vi "Display Menu.vi"(8 "Startup Menu?(F)":bool, 9 "Display Rules?(F)":bool, 10 "Reference In":refnum<vi>, 11 "Internal Data In":T1) -> (3 "Internal a Out":T1)   [LabVIEW 2025]
uses:
  Internal Data.ctl
  Collision Box.ctl
  <vilib>/picture/picture.llb/imagedata.ctl
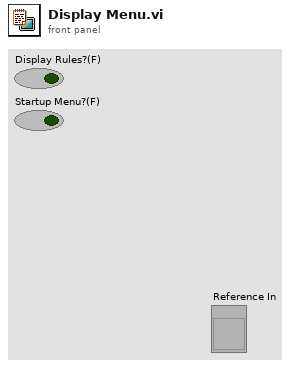
[diagram p1: front panel]
types:
  T1 = typedef "Internal Data.ctl" = cluster{"Core":cluster{"Current VI Reference":refnum<vi>, "Close Panel on Exit?":bool}, "Collision Box":T2, "Walls":cluster{"[0]":T3, "[1]":T3, "[2]":T3, "[3]":T3, "[4]":T3, "[5]":T3, "[6]":T3, "[7]":T3, "[8]":T3}, "Floor":T3, "Gates":cluster{"[0]":T3, "[1]":T3, "[2]":T3, "[3]":T3, "[4]":T3, "[5]":T3, "[6]":T3, "[7]":T3, "[8]":T3}, "Gate Condition":bool[], "Level":i32, "Score":i32, "Player Image":T3, "Display Font":cluster{"Font Name:":string, "Size":i16, "Strikeout?":bool, "Italic?":bool, "Underline?":bool, "Outline?":bool, "Shadow?":bool, "Bold?":bool}, "Menu Image":T3, "Menu Button Image":T3, "Menu Selected Image":T3, "Menu Selection":i32, "Player Name":string, "Menu Wall Image":T3}
  T2 = typedef "Collision Box.ctl" = cluster{"left":i16, "top":i16, "right":i16, "bottom":i16}
  T3 = typedef "imagedata.ctl" = cluster{"image type":i32, "image depth":i32, "image":u8[], "mask":u8[], "colors":u32[], "Rectangle":cluster{"left":i16, "top":i16, "right":i16, "bottom":i16}}
  T4 = enum16{"User-specified Font", "Application Font", "System Font", "Dialog Font"}
  T5 = cluster{"left":i16, "top":i16, "right":i16, "bottom":i16}
  T6 = cluster{"horizontal":enum16{"left", "center", "right"}, "vertical":enum16{"top", "center", "bottom"}}
  T7 = cluster{"Font Name:":string, "Size":i16, "Strikeout?":bool, "Italic?":bool, "Underline?":bool, "Outline?":bool, "Shadow?":bool, "Bold?":bool}
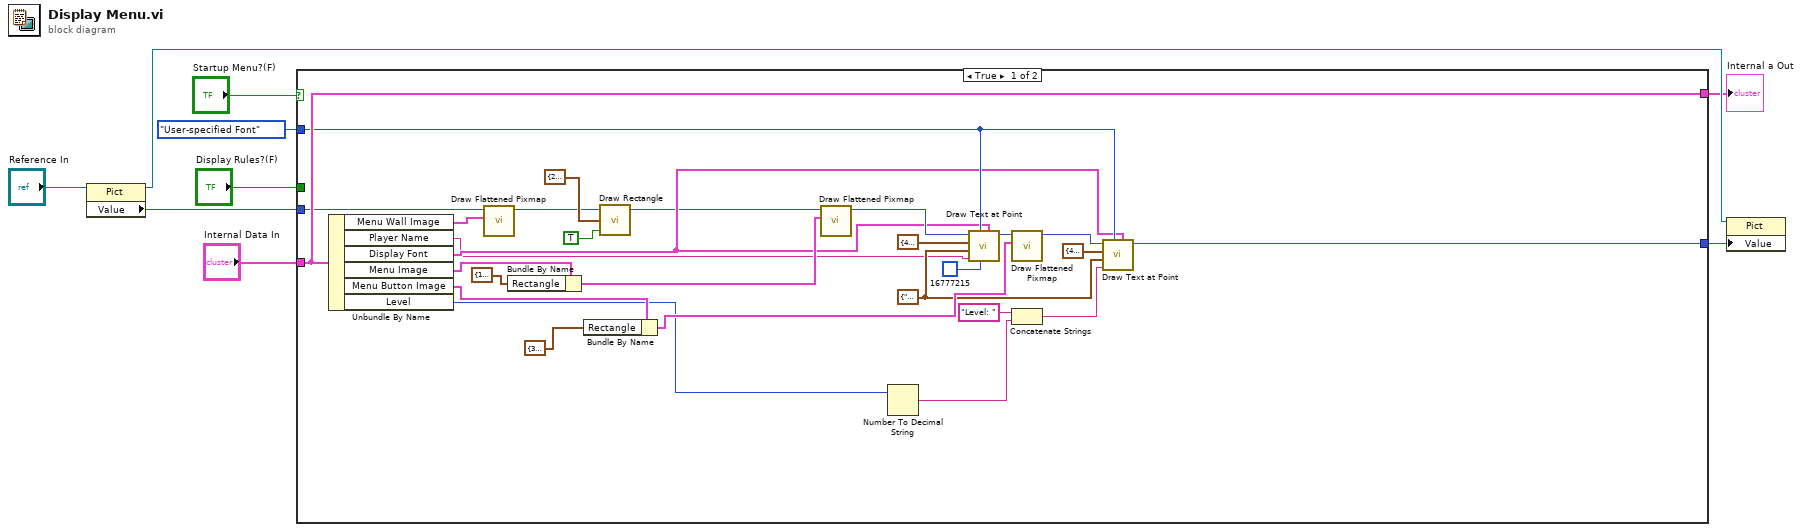
[diagram p0: block diagram]
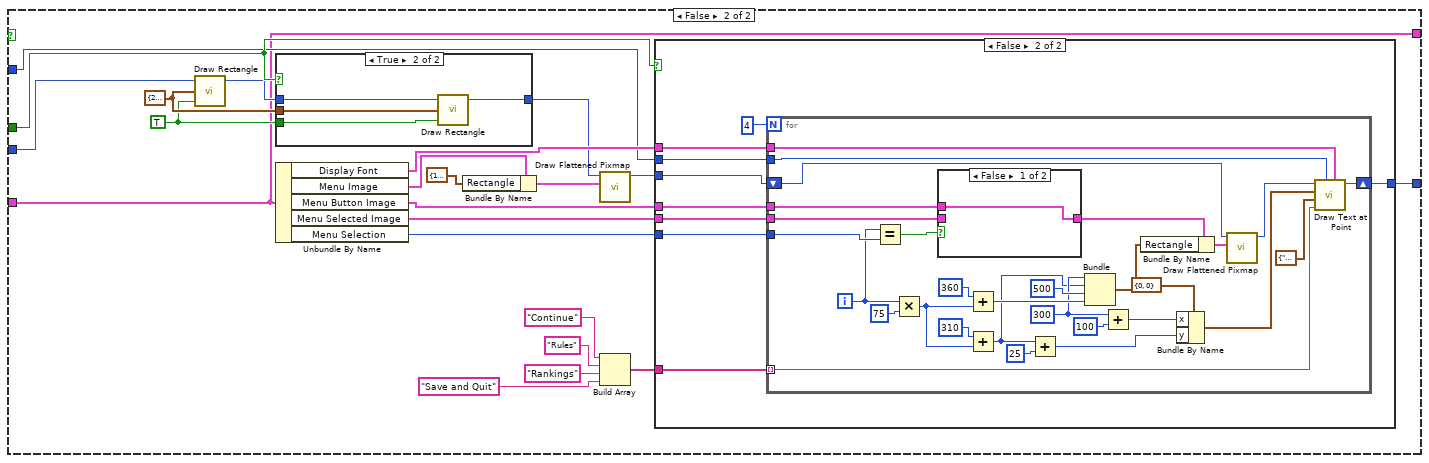
[diagram p2: hidden frame]
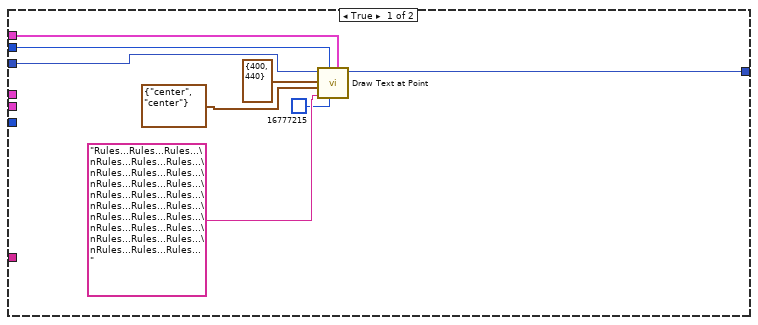
[diagram p3: hidden frame]
diagram:
  n1 = property on="Property Node" class="Pict"(reference="Reference In") -> (reference out=w7:refnum<vi>, "Value"=w6:picture)  [unwired: 1 in, 1 out]
  n2 = case shown="True" "Startup Menu?(F)" {
    tunnel: [w25 w53] -> w9
    tunnel: w6 -> [w15 w51]
    tunnel: "Display Rules?(F)" -> [_ w49]
    tunnel: "Internal Data In" -> [w34 w38]
    tunnel: [w34 w38] -> w1
    tunnel: T4."User-specified Font" ("desired font(Application)") -> [w24 w44]
    frame True {
      w22 = T6 {"horizontal"=enum."center", "vertical"=enum."center"} ("alignment(left, top)")
      n3 = Unbundle By Name(w34) -> ("Menu Wall Image"=w14:T3, "Player Name"=w16:string, "Display Font"=w23:T7, "Menu Image"=w36:T3, "Menu Button Image"=w32:T3, "Level"=w20:i32)
      n4 = call <vilib>:"Draw Flattened Pixmap.vi"("image data"=w14, "picture"=w15) -> ("new picture"=w11:picture)  [unwired: 7 in]
      n5 = Bundle By Name(cluster=w36, "Rectangle"=T5 {"left"=150, "top"=300, "right"=650, "bottom"=815}) -> (w35:T3)
      n6 = Bundle By Name(cluster=w32, "Rectangle"=T5 {"left"=300, "top"=600, "right"=500, "bottom"=650}) -> (w31:T3)
      n7 = call <vilib>:"Draw Rectangle.vi"("picture"=w11, "rect"=T5 {"left"=200, "top"=350, "right"=600, "bottom"=800} ("Rectangle"), "fill?(F)"=TRUE) -> ("new picture"=w10:picture)  [unwired: 6 in]
      n8 = call <vilib>:"Draw Flattened Pixmap.vi"("image data"=w35, "picture"=w10) -> ("new picture"=w30:picture)  [unwired: 7 in]
      n9 = Number To Decimal String(number=w20) -> (decimal integer string=w19:string)  [unwired: 1 in]
      n10 = call <vilib>:"Draw Text at Point.vi"("[user-specified font]"=w23, "text color(black)"=u32 16777215, "desired font(Application)"=w24, "text"=w16, "alignment(left, top)"=w22, "origin"=cluster{"x":i16, "y":i16} {"x"=400, "y"=550}, "picture"=w30) -> ("new picture"=w29:picture)  [unwired: 3 in, 1 out]
      n11 = call <vilib>:"Draw Flattened Pixmap.vi"("image data"=w31, "picture"=w29) -> ("new picture"=w26:picture)  [unwired: 7 in]
      n12 = Concatenate Strings("Level: " ("string"), w19) -> (w17:string)
      n13 = call <vilib>:"Draw Text at Point.vi"("[user-specified font]"=w23, "desired font(Application)"=w24, "text"=w17, "alignment(left, top)"=w22, "origin"=cluster{"x":i16, "y":i16} {"x"=400, "y"=625}, "picture"=w26) -> ("new picture"=w25:picture)  [unwired: 4 in, 1 out]
    }
    frame False {
      w45 = TRUE ("fill?(F)")
      w46 = T5 {"left"=200, "top"=200, "right"=600, "bottom"=650} ("Rectangle")
      n14 = call <vilib>:"Draw Rectangle.vi"("picture"=w51, "rect"=w46, "fill?(F)"=w45) -> ("new picture"=w48:picture)  [unwired: 6 in]
      n15 = case shown="True" w49 {
        tunnel: w48 -> [w108 w112]
        tunnel: [w108 w111] -> w47
        tunnel: w46 -> [_ w110]
        tunnel: w45 -> [_ w109]
        frame False {
        }
        frame True {
          n16 = call <vilib>:"Draw Rectangle.vi"("picture"=w112, "rect"=w110, "fill?(F)"=w109) -> ("new picture"=w111:picture)  [unwired: 6 in]
        }
      }
      n17 = Unbundle By Name(w38) -> ("Display Font"=w54:T7, "Menu Image"=w57:T3, "Menu Button Image"=w56:T3, "Menu Selected Image"=w55:T3, "Menu Selection"=w52:i32)
      n18 = Bundle By Name(cluster=w57, "Rectangle"=T5 {"left"=150, "top"=150, "right"=650, "bottom"=665}) -> (w59:T3)
      n19 = call <vilib>:"Draw Flattened Pixmap.vi"("image data"=w59, "picture"=w47) -> ("new picture"=w58:picture)  [unwired: 7 in]
      n20 = Build Array("Continue" ("element"), "Rules" ("element"), "Rankings" ("element"), "Save and Quit") -> (w39:string[])
      n21 = case shown="False" w49 {
        tunnel: w58 -> [w67 w76]
        tunnel: w56 -> [_ w75]
        tunnel: w55 -> [_ w73]
        tunnel: w54 -> [w64 w72]
        tunnel: [w66 w71] -> w53
        tunnel: w52 -> [_ w70]
        tunnel: w44 -> [w65 w69]
        tunnel: w39 -> [_ w68]
        frame True {
          n22 = call <vilib>:"Draw Text at Point.vi"("[user-specified font]"=w64, "text color(black)"=u32 16777215, "desired font(Application)"=w65, "text"="Rules...Rules...Rules...\nRules...Rules...Rules...\nRules...Rules...Rules...\nRules...Rules...Rules...\nRules...Rules...Rules...\nRules...Rules...Rules...\nRules...Rules...Rules...\nRules...Rules...Rules...\nRules...Rules...Rules...\nRules...Rules...Rules...", "alignment(left, top)"=T6 {"horizontal"=enum."center", "vertical"=enum."center"}, "origin"=cluster{"x":i16, "y":i16} {"x"=400, "y"=440}, "picture"=w67) -> ("new picture"=w66:picture)  [unwired: 3 in, 1 out]
        }
        frame False {
          n23 = for {
            N: 4 -> [_]
            tunnel: w75 -> [w98]
            shift-right: [w92] -> w71
            shift-left: w76 -> [w105]
            tunnel: w73 -> [w97]
            tunnel: w68 -> [w90] mode=indexing
            tunnel: w72 -> [w91]
            tunnel: w70 -> [w80]
            tunnel: w69 -> [w77]
            i -> [w79]
            w86 = i16 300 ("left")
            n24 = Equal?(x=w79, y=w80) -> (x = y?=w78:bool)
            n25 = Multiply(x=w79, y=75) -> (x*y=w100:i32)
            n26 = case shown="False" w78 {
              tunnel: w98 -> [w106 _]
              tunnel: w97 -> [_ w107]
              tunnel: [w106 w107] -> w95
              frame False {
              }
              frame True {
              }
            }
            n27 = Add(x=360 ("bottom"), y=w100) -> (x+y=w99:i32)
            n28 = Add(x=310 ("top"), y=w100) -> (x+y=w83:i32)
            n29 = Add(x=w83, y=25) -> (x+y=w81:i32)
            n30 = Bundle("left"=w86, w83, "right"=i16 500, w99) -> (w94:cluster{"left":i16, i32, "right":i16, i32})  [unwired: 1 in]
            n31 = Add(x=w86, y=i16 100) -> (x+y=w84:i16)
            n32 = Bundle By Name(cluster=w95, "Rectangle"=w94) -> (w96:T3)
            n33 = Bundle By Name(cluster=cluster{"x":i16, "y":i16} {"x"=0, "y"=0} ("origin"), "x"=w84, "y"=w81) -> (w87:cluster{"x":i16, "y":i16})
            n34 = call <vilib>:"Draw Flattened Pixmap.vi"("image data"=w96, "picture"=w105) -> ("new picture"=w93:picture)  [unwired: 7 in]
            n35 = call <vilib>:"Draw Text at Point.vi"("[user-specified font]"=w91, "desired font(Application)"=w77, "text"=w90, "alignment(left, top)"=T6 {"horizontal"=enum."center", "vertical"=enum."center"}, "origin"=w87, "picture"=w93) -> ("new picture"=w92:picture)  [unwired: 4 in, 1 out]
          }
        }
      }
    }
  }
  "Internal a Out" <- w1
  n36 = property on="Property Node" class="Pict"(reference=w7, "Value"=w9) -> ()  [unwired: 1 in, 2 out]
